vi "save_xml.vi"(8 "error in (no error)":errorcluster, 9 "appended path":path, 10 "string":string, 11 "DataCollectionDL110128Streaming in":refnum<class "DataCollectionDL110128Streaming.lvclass">) -> (0 "error out":errorcluster, 3 "DataCollectionDL110128Streaming out":refnum<class "DataCollectionDL110128Streaming.lvclass">)   [LabVIEW 2010, in "DataCollectionDL110128Streaming.lvclass"]
uses:
  DataCollectionDL110128Streaming.lvclass
  common/classes/XMLElement/XMLElement/XMLElement.lvclass
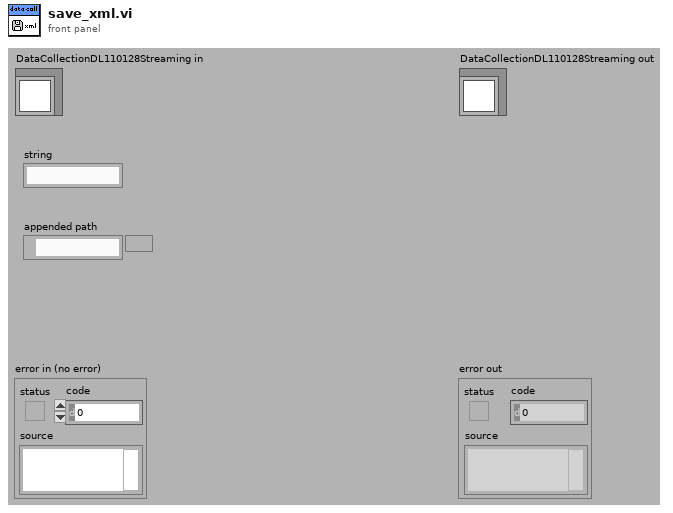
[diagram p1: front panel]
types:
  T1 = enum16{"open", "replace", "create", "open or create", "replace or create", "replace or create with confirmation"}
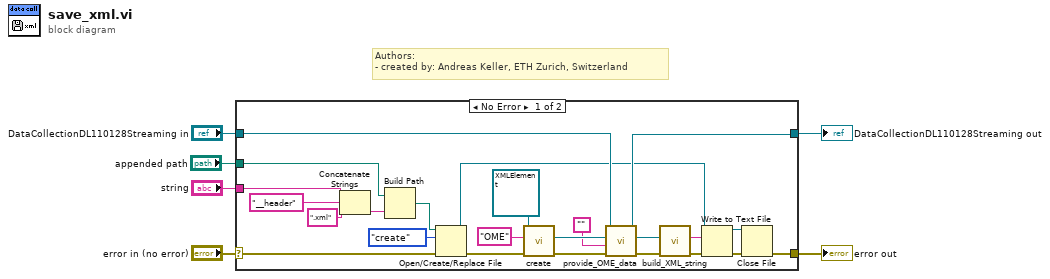
[diagram p0: block diagram]
diagram:
  # "Authors: \n- created by: Andreas Keller, ETH Zurich, Switzerland"
  n1 = case shown="No Error" "error in (no error)" {
    selector: "error in (no error)" -> [w23 w32]
    tunnel: [w21 w32] -> w5
    tunnel: [w13 w31] -> w3
    tunnel: "DataCollectionDL110128Streaming in" -> [w14 w31]
    tunnel: "string" -> [w26 _]
    tunnel: "appended path" -> [w25 _]
    frame No Error {
      n2 = Concatenate Strings(w26, "__header", ".xml") -> (w29:string)
      n3 = Build Path(base path=w25, name or relative path=w29) -> (appended path=w24:path)
      n4 = Open/Create/Replace File(file path (use dialog)=w24, error in=w23, operation (0:open)=T1."create") -> (refnum out=w7:refnum<file>, error out=w9:errorcluster)  [unwired: 3 in, 1 out]
      n5 = call "create.vi"("error in (no error)"=w9, "name"="OME", "XMLElement in"=refnum<class "XMLElement.lvclass"> refnum ("XMLElement.lvclass")) -> ("error out"=w16:errorcluster, "XMLElement out"=w17:refnum<class "XMLElement.lvclass">)  [unwired: 7 in]
      n6 = call-dynamic "provide_OME_data.vi"("error in (no error)"=w16, "structuredAttribute string in"="", "OME element in"=w17, "DataCollectionDL091104Scaffold in"=w14) -> ("error out"=w11:errorcluster, "OME element out"=w12:refnum<class "XMLElement.lvclass">, "DataCollectionDL091104Scaffold out"=w13:refnum<class "DataCollectionDL110128Streaming.lvclass">)  [unwired: 4 in, 1 out]
      n7 = call "build_XML_string.vi"("error in (no error)"=w11, "Element in"=w12) -> ("error out"=w8:errorcluster, "string"=w10:string)  [unwired: 7 in, 1 out]
      n8 = Write to Text File(file (use dialog)=w7, text=w10, error in=w8) -> (refnum out=w20:refnum<file>, error out=w22:errorcluster)  [unwired: 1 in, 1 out]
      n9 = Close File(refnum=w20, error in=w22) -> (error out=w21:errorcluster)  [unwired: 1 out]
    }
    frame Error {
    }
  }
  "error out" <- w5
  "DataCollectionDL110128Streaming out" <- w3
